vi "Shutdown1.vi"(8 "error in (no error)":errorcluster, 11 "device data model in":refnum<class "Standard Data Model1.lvclass">) -> (0 "error out":errorcluster)   [LabVIEW 2019, in "NI_modbus_upd.lvlib" / "Standard Data Model1.lvclass"]
doc: "This VI is responsible for deleting the device data model."
uses:
  Standard Data Model1.lvclass
  Standard Data Model1.lvclass/Standard Data Model1.ctl
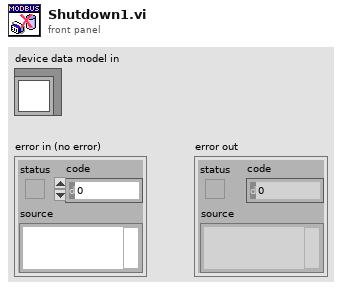
[diagram p1: front panel]
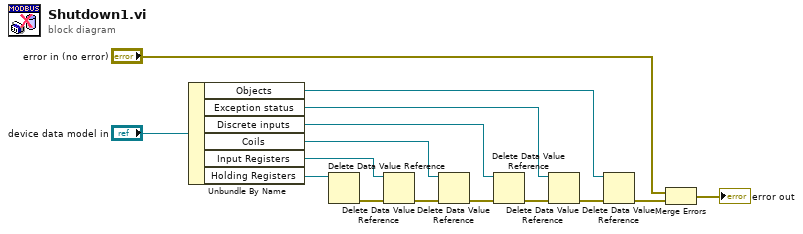
[diagram p0: block diagram]
diagram:
  n1 = Unbundle By Name("device data model in") -> ("Objects"=w5:refnum<data-value>, "Exception status"=w4:refnum<data-value>, "Discrete inputs"=w14:refnum<data-value>, "Coils"=w13:refnum<data-value>, "Input Registers"=w12:refnum<data-value>, "Holding Registers"=w11:refnum<data-value>)
  n2 = Delete Data Value Reference(data value reference=w11) -> (error out=w10:errorcluster)  [unwired: 1 in, 1 out]
  n3 = Delete Data Value Reference(data value reference=w12, error in=w10) -> (error out=w9:errorcluster)  [unwired: 1 out]
  n4 = Delete Data Value Reference(data value reference=w13, error in=w9) -> (error out=w8:errorcluster)  [unwired: 1 out]
  n5 = Delete Data Value Reference(data value reference=w14, error in=w8) -> (error out=w6:errorcluster)  [unwired: 1 out]
  n6 = Delete Data Value Reference(data value reference=w4, error in=w6) -> (error out=w7:errorcluster)  [unwired: 1 out]
  n7 = Delete Data Value Reference(data value reference=w5, error in=w7) -> (error out=w2:errorcluster)  [unwired: 1 out]
  n8 = Merge Errors("error in (no error)", w2) -> (→"error out":errorcluster)
